vi "Test_Read_Light_Team072.vi"() -> ()   [LabVIEW 2016]
panel:
  in  "Color Sensing Mode":string(combo)
  out "Average Measurement Value":dbl
  in  "Number of Measurements to Take":dbl
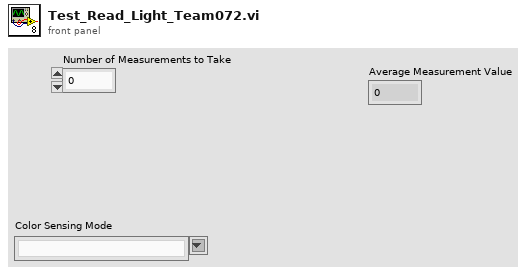
[diagram p1: front panel]
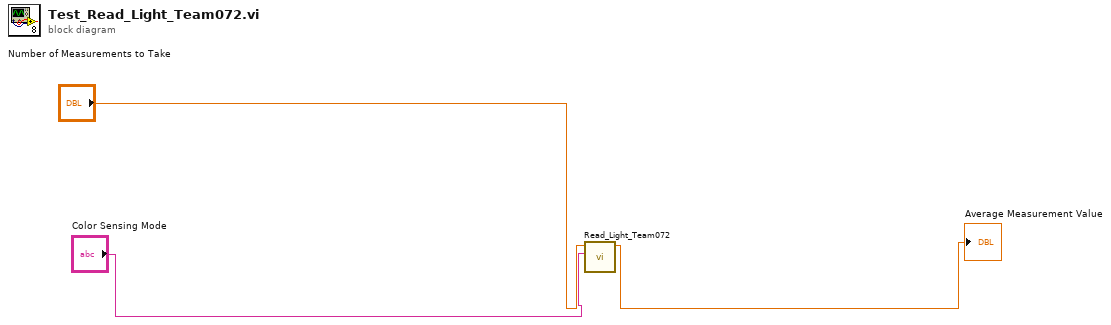
[diagram p0: block diagram]
diagram:
  n1 = call "Read_Light_Team072.vi"("Color Sensing Mode"="Color Sensing Mode", "Number of Measurements to Take"="Number of Measurements to Take") -> ("Average Measurement Value"=→"Average Measurement Value":dbl)  [unwired: 9 in]
